vi "NI VeriStand - Read Single Waveform (DBL).vi"(8 "error in (no error)":errorcluster, 10 "timeout in ms (-1)":i32=-1, 11 "Single Waveform Read Session (DBL) in":refnum<class "Single Waveform Read (DBL).lvclass">) -> (0 "error out":errorcluster, 1 "Properties":T1, 2 "Data":dbl[](array[numeric]), 3 "Single Waveform Read Session (DBL) out":refnum<class "Single Waveform Read (DBL).lvclass">, 4 "timed out?":bool)   [LabVIEW 2020, in "NI_VS Custom Device Waveform API.lvlib" / "Single Waveform Read (DBL).lvclass"]
doc: "Reads data from a waveform(s) associated with the specified read session."
uses:
  Single Waveform Read (DBL).lvclass
  D:/p4/penguin/lvaddon/Veristand/master/src/LabVIEW/vilib/NI VeriStand/Custom Device Waveform API/Waveform Session.lvclass
  Waveform properties.ctl
  Custom Device API/Waveform Data Reference.ctl
  Waveform Session.lvclass/Waveform Session.ctl
  Single Waveform Read (DBL).lvclass/Single Waveform Read (DBL).ctl
  Internal Comm Classes/WPL Comm/WPL Comm (1D DBL)/WPL Comm (1D DBL).lvclass/WPL Comm (1D DBL).ctl
  Internal Comm Classes/WPL Comm/Convert Q Error to Shutdown Error.vi
  <vilib>/Utility/error.llb/Error Cluster From Error Code.vi
  Internal Comm Classes/WPL Comm/WPL Comm (1D DBL)/WPL Comm (1D DBL).lvclass
  Waveform Session.lvclass
  NI_VS Custom Device Waveform API.lvlib
  Custom Device API/Custom Device API.lvlib
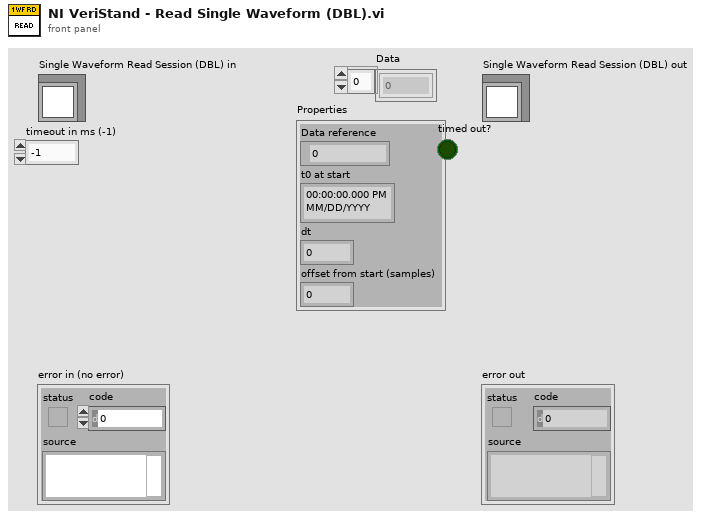
[diagram p1: front panel]
types:
  T1 = typedef "NI_VS Custom Device Waveform API.lvlib/Waveform properties.ctl" = cluster{"Data reference":T2, "t0 at start":timestamp, "dt":dbl, "offset from start (samples)":u64}
  T2 = typedef "Custom Device API.lvlib/Waveform Data Reference.ctl" = i32
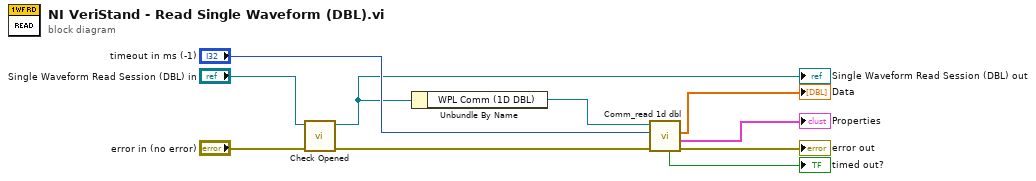
[diagram p0: block diagram]
diagram:
  n1 = call "Check Opened.vi"("error in (no error)"="error in (no error)", "Waveform Session in"="Single Waveform Read Session (DBL) in") -> ("error out"=w6:errorcluster, "Waveform Session out"=w4:refnum<class "Single Waveform Read (DBL).lvclass">)  [unwired: 8 in]
  "Single Waveform Read Session (DBL) out" <- w4
  n2 = Unbundle By Name(w4) -> ("WPL Comm (1D DBL)"=w3:refnum<class "WPL Comm (1D DBL).lvclass">)
  n3 = call "Comm_read 1d dbl.vi"("error in (no error)"=w6, "timeout in ms (-1)"="timeout in ms (-1)", "WPL Comm (1D DBL) in"=w3) -> ("error out"=→"error out":errorcluster, "Properties"=→"Properties":T1, "Data"=→"Data":dbl[], "timed out?"=→"timed out?":bool)  [unwired: 5 in]
